vi "No Load Condition.vi"() -> (1 "String for Log":string, 2 "Data out":dbl[](array[numeric]), 3 "Report Cell Names":string[](array[string]))   [LabVIEW 2018]
uses:
  Globals/Data Globals.vi
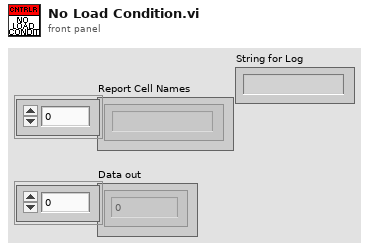
[diagram p1: front panel]
types:
  T1 = typedef "All Data Cluster.ctl" = cluster{"Acq Data":T2, "Post-Analysis Data":T3}
  T2 = typedef "Acq Data.ctl" = cluster{"Timestamp":timestamp, "Acq Period (ms)":i64, "00-00-9205":dbl[], "00-01-9205":dbl[], "01-00-9213":dbl[], "01-01-9213":dbl[], "01-02-9213":dbl[], "02-02-9219":dbl[], "02-03-9227":dbl[], "00-02-9234 Raw":dbl[], "00-02-9234 DC":dbl[], "00-02-9234 RMS":dbl[], "00-02-9234 Peak":dbl[], "00-02-9234 Freq":dbl[], "00-03-9402":dbl[], "02-05-9205":dbl[], "02-04-9871":dbl[]}
  T3 = typedef "Post-Analysis Data.ctl" = cluster{"Calibrated Data":cluster{"00-00-9205 Calib":dbl[], "00-01-9205 Calib":dbl[], "01-00-9213 Calib":dbl[], "01-01-9213 Calib":dbl[], "01-02-9213 Calib":dbl[], "02-02-9219 Calib":dbl[], "02-03-9227 Calib":dbl[], "00-02-9234 Calib":dbl[], "00-03-9402 Calib":dbl[], "02-05-9205 Calib":dbl[], "02-04-9871 2DArray":dbl[][]}, "Calculated Data":T4, "Indicator Data":cluster{"00-02-9234 Power Spectras":cluster{"z0":dbl, "dz":dbl, "waveforms":cluster{"f0":dbl, "df":dbl, "magnitude":dbl[]}[]}[], "00-02-9234 Peak Vel (in/sec)":dbl[], "Interactive Mode Vals":dbl[]}}
  T4 = typedef "Calculated Data.ctl" = cluster{"C.00":dbl, "C.01":dbl, "C.02":dbl, "C.03":dbl, "C.04":dbl, "C.05":dbl, "C.06":dbl, "C.07":dbl, "C.08":dbl, "C.09":dbl, "C.10":dbl, "C.11":dbl, "C.12":dbl, "C.13":dbl, "C.14":dbl, "C.15":dbl, "C.16":dbl, "C.17":dbl, "C.18":dbl, "C.19":dbl, "C.20":dbl, "C.21":dbl, "C.22":dbl, "C.23":dbl, "C.24":dbl, "C.25":dbl, "C.26":dbl, "C.27":dbl, "C.28":dbl, "C.29":dbl, "C.30":dbl, "C.31":dbl, "C.32":dbl, "C.33":dbl, "C.34":dbl, "C.35":dbl, "C.36":dbl, "C.37":dbl, "C.38":dbl, "C.39":dbl, "C.40":dbl, "C.41":dbl, "C.42":dbl, "C.43":dbl, "C.44":dbl, "C.45":dbl, "C.46":dbl, "C.47":dbl, "C.48":dbl, "C.49":dbl, "C.50":dbl, "C.51":dbl, "C.52":dbl, "C.53":dbl, "C.54":dbl, "C.56":dbl}
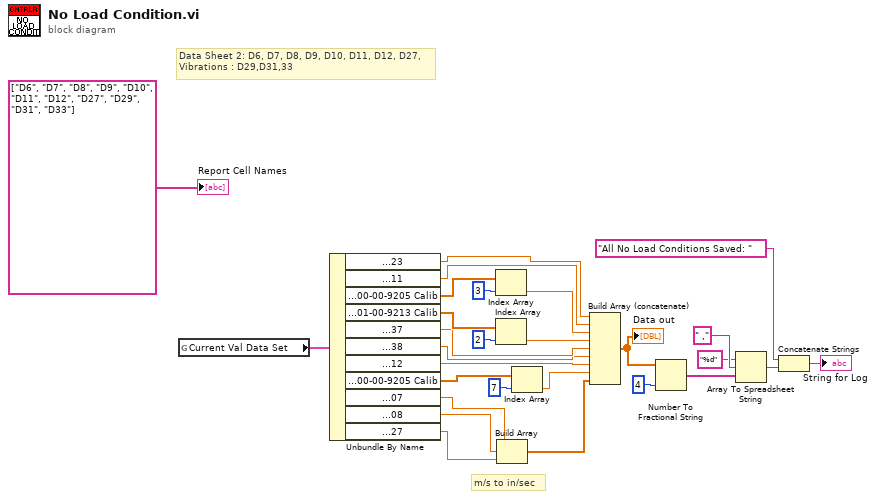
[diagram p0: block diagram]
diagram:
  # "m/s to in/sec"
  # "Data Sheet 2: D6, D7, D8, D9, D10, D11, D12, D27, \nVibrations : D29,D31,33"
  n1 = global read "Data Globals.vi" "Current Val Data Set"() -> (w18:T1)
  n2 = Unbundle By Name(w18) -> ("Post-Analysis Data.Calculated Data.C.23"=w5:dbl, "Post-Analysis Data.Calculated Data.C.11"=w28:dbl, "Post-Analysis Data.Calibrated Data.00-00-9205 Calib"=w27:dbl[], "Post-Analysis Data.Calibrated Data.01-00-9213 Calib"=w23:dbl[], "Post-Analysis Data.Calculated Data.C.37"=w21:dbl, "Post-Analysis Data.Calculated Data.C.38"=w20:dbl, "Post-Analysis Data.Calculated Data.C.12"=w19:dbl, "Post-Analysis Data.Calibrated Data.00-00-9205 Calib"=w17:dbl[], "Post-Analysis Data.Calculated Data.C.07"=w4:dbl, "Post-Analysis Data.Calculated Data.C.08"=w3:dbl, "Post-Analysis Data.Calculated Data.C.27"=w2:dbl)
  n3 = Index Array(array=w27, index=3) -> (element=w25:dbl)
  n4 = Index Array(array=w23, index=2) -> (element=w22:dbl)
  n5 = Build Array(w4, w3, w2) -> (w1:dbl[])
  n6 = Index Array(array=w17, index=7) -> (element=w15:dbl)
  n7 = Build Array (concatenate)(w5, w28, w25, w22, w21, w20, w19, w15, w1) -> (w11:dbl[])
  "Data out" <- w11
  n8 = Number To Fractional String(number=w11, precision (6)=i16 4) -> (F-format string=w13:string[])  [unwired: 2 in]
  n9 = Array To Spreadsheet String(delimiter (Tab)=" ,", array=w13, 3:"%d" ("format string")) -> (spreadsheet string=w8:string)
  n10 = Concatenate Strings("All No Load Conditions Saved: " ("Message"), w8) -> (→"String for Log":string)
  "Report Cell Names" <- string[] ["D6", "D7", "D8", "D9", "D10", "D11", "D12", "D27", "D29", "D31", "D33"] ("array w/ subset deleted")
